vi "HLEN.vi"(8 "error in (no error)":errorcluster, 10 "key":string, 11 "Redis Client in":refnum<class "Redis Client.lvclass">) -> (0 "error out":errorcluster, 1 "# of fields":i64, 3 "Redis Client out":refnum<class "Redis Client.lvclass">)   [LabVIEW 2019, in "Redis Client for LabVIEW.lvlib" / "Redis Client.lvclass"]
uses:
  Redis Client.lvclass
  lib/RESP3-for-LabVIEW/RESP3/subVIs/RESP3 Make String Base.vi
  lib/RESP3-for-LabVIEW/RESP3/types/RESP3 data type attribute.vi
  lib/RESP3-for-LabVIEW/RESP3/high-level/RESP3 Get String.vi
  lib/RESP3-for-LabVIEW/RESP3/RESP3.lvlib
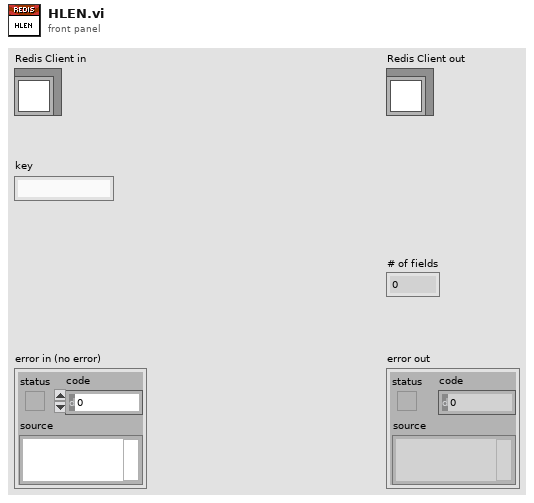
[diagram p1: front panel]
types:
  T1 = typedef "RESP3.lvlib/RESP3 Type.ctl" = enum8{"<0x00>", "<0x01>", "<0x02>", "<0x03>", "<0x04>", "<0x05>", "<0x06>", "<0x07>", "<0x08>", "<0x09>", "<0x0A>", "<0x0B>", "<0x0C>", "<0x0D>", "<0x0E>", "<0x0F>", "<0x10>", "<0x11>", "<0x12>", "<0x13>", "<0x14>", "<0x15>", "<0x16>", "<0x17>", "<0x18>", "<0x19>", "<0x1A>", "<0x1B>", "<0x1C>", "<0x1D>", "<0x1E>", "<0x1F>", "\" \"", "BLOB ERROR", "\"\"\"", "BOOLEAN", "BLOB", "MAP", "\"&\"", "\"'\"", "BIG NUMBER", "\")\"", "ARRAY", "STRING", "DOUBLE", "ERROR", "END", "\"/\"", "\"0\"", "\"1\"", "\"2\"", "\"3\"", "\"4\"", "\"5\"", "\"6\"", "\"7\"", "\"8\"", "\"9\"", "INTEGER", "STREAM", "\"<\"", "VERBATIM STRING", "PUSH", "\"?\"", "\"@\"", "\"A\"", "\"B\"", "\"C\"", "\"D\"", "\"E\"", "\"F\"", "\"G\"", "\"H\"", "\"I\"", "\"J\"", "\"K\"", "\"L\"", "\"M\"", "\"N\"", "\"O\"", "\"P\"", "\"Q\"", "\"R\"", "\"S\"", "\"T\"", "\"U\"", "\"V\"", "\"W\"", "\"X\"", "\"Y\"", "\"Z\"", "\"[\"", "\"\\\"", "\"]\"", "\"^\"", "NULL", "\"`\"", "\"a\"", "\"b\"", "\"c\"", "\"d\"", "\"e\"", "\"f\"", "\"g\"", "\"h\"", "\"i\"", "\"j\"", "\"k\"", "\"l\"", "\"m\"", "\"n\"", "\"o\"", "\"p\"", "\"q\"", "\"r\"", "\"s\"", "\"t\"", "\"u\"", "\"v\"", "\"w\"", "\"x\"", "\"y\"", "\"z\"", "\"{\"", "ATTRIBUTES", "\"}\"", "SET", "<0x7F>", "<0x80>", "<0x81>", "<0x82>", "<0x83>", "<0x84>", "<0x85>", "<0x86>", "<0x87>", "<0x88>", "<0x89>", "<0x8A>", "<0x8B>", "<0x8C>", "<0x8D>", "<0x8E>", "<0x8F>", "<0x90>", "<0x91>", "<0x92>", "<0x93>", "<0x94>", "<0x95>", "<0x96>", "<0x97>", "<0x98>", "<0x99>", "<0x9A>", "<0x9B>", "<0x9C>", "<0x9D>", "<0x9E>", "<0x9F>", "<0xA0>", "<0xA1>", "<0xA2>", "<0xA3>", "<0xA4>", "<0xA5>", "<0xA6>", "<0xA7>", "<0xA8>", "<0xA9>", "<0xAA>", "<0xAB>", "<0xAC>", "<0xAD>", "<0xAE>", "<0xAF>", "<0xB0>", "<0xB1>", "<0xB2>", "<0xB3>", "<0xB4>", "<0xB5>", "<0xB6>", "<0xB7>", "<0xB8>", "<0xB9>", "<0xBA>", "<0xBB>", "<0xBC>", "<0xBD>", "<0xBE>", "<0xBF>", "<0xC0>", "<0xC1>", "<0xC2>", "<0xC3>", "<0xC4>", "<0xC5>", "<0xC6>", "<0xC7>", "<0xC8>", "<0xC9>", "<0xCA>", "<0xCB>", "<0xCC>", "<0xCD>", "<0xCE>", "<0xCF>", "<0xD0>", "<0xD1>", "<0xD2>", "<0xD3>", "<0xD4>", "<0xD5>", "<0xD6>", "<0xD7>", "<0xD8>", "<0xD9>", "<0xDA>", "<0xDB>", "<0xDC>", "<0xDD>", "<0xDE>", "<0xDF>", "<0xE0>", "<0xE1>", "<0xE2>", "<0xE3>", "<0xE4>", "<0xE5>", "<0xE6>", "<0xE7>", "<0xE8>", "<0xE9>", "<0xEA>", "<0xEB>", "<0xEC>", "<0xED>", "<0xEE>", "<0xEF>", "<0xF0>", "<0xF1>", "<0xF2>", "<0xF3>", "<0xF4>", "<0xF5>", "<0xF6>", "<0xF7>", "<0xF8>", "<0xF9>", "<0xFA>", "<0xFB>", "<0xFC>", "<0xFD>", "<0xFE>"}
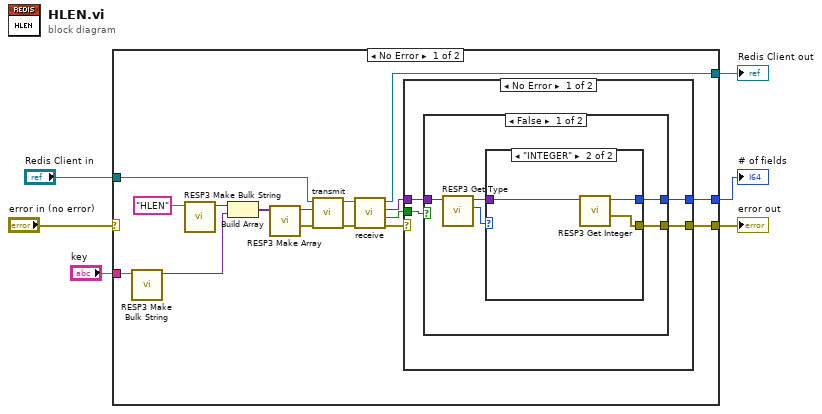
[diagram p0: block diagram]
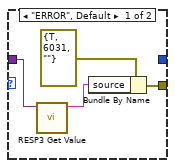
[diagram p2: hidden frame]
diagram:
  n1 = case shown="No Error" "error in (no error)" {
    selector: "error in (no error)" -> [_ w41]
    tunnel: [w14 w41] -> w5
    tunnel: "Redis Client in" -> [w22 w40]
    tunnel: [w19 w40] -> w3
    tunnel: "key" -> [w11 _]
    tunnel: [w13 _] -> w1
    frame No Error {
      n2 = call "RESP3 Make Bulk String.vi"("String"=w11) -> ("RESP3 Value out"=w9:variant)  [unwired: 9 in, 1 out]
      n3 = call "RESP3 Make Bulk String.vi"("String"="HLEN" ("string in")) -> ("RESP3 Value out"=w10:variant)  [unwired: 9 in, 1 out]
      n4 = Build Array(w10, w9) -> (w21:variant[])
      n5 = call "RESP3 Make Array.vi"("RESP3 Values in"=w21) -> ("error out"=w8:errorcluster, "RESP3 Value out"=w7:variant)  [unwired: 9 in]
      n6 = call-dynamic "transmit.vi"("error in (no error)"=w8, "RESP3 Value"=w7, "Redis Client in"=w22) -> ("error out"=w18:errorcluster, "Redis Client out"=w20:refnum<class "Redis Client.lvclass">)  [unwired: 7 in]
      n7 = call-dynamic "receive.vi"("error in (no error)"=w18, "Redis Client in"=w20) -> ("error out"=w17:errorcluster, "timed out?"=w16:bool, "RESP3 Value"=w15:variant, "Redis Client out"=w19:refnum<class "Redis Client.lvclass">)  [unwired: 6 in]
      n8 = case shown="No Error" w17 {
        selector: w17 -> [_ w39]
        tunnel: [w26 _] -> w13
        tunnel: [w25 w39] -> w14
        tunnel: w15 -> [w23 _]
        tunnel: w16 -> [w24 _]
        frame No Error {
          n9 = case shown="False" w24 {
            tunnel: [w31 _] -> w26
            tunnel: [w30 _] -> w25
            tunnel: w23 -> [w29 _]
            frame False {
              n10 = call "RESP3 Get Type.vi"("RESP3 Value in"=w29) -> ("RESP3 Type"=w27:T1, "RESP3 Value out"=w28:variant)  [unwired: 7 in, 2 out]
              n11 = case shown="\"INTEGER\"" w27 {
                tunnel: [_ w38] -> w31
                tunnel: [w34 w37] -> w30
                tunnel: w28 -> [w33 w36]
                frame "ERROR", Default {
                  n12 = call-poly "RESP3 Get Value.vi"("RESP3 Value in"=w33) -> ("String out"=w32:string)  [unwired: 7 in, 3 out]
                  n13 = Bundle By Name(cluster=errorcluster {"status"=TRUE, "code"=6031, "source"=""} ("error constant"), "source"=w32) -> (w34:errorcluster)
                }
                frame "INTEGER" {
                  n14 = call "RESP3 Get Integer.vi"("RESP3 Value in"=w36) -> ("error out"=w37:errorcluster, "I64 out"=w38:i64)  [unwired: 8 in, 1 out]
                }
              }
            }
            frame True {
            }
          }
        }
        frame Error {
        }
      }
    }
    frame Error {
    }
  }
  "error out" <- w5
  "Redis Client out" <- w3
  "# of fields" <- w1
